vi "generate cartesian circle points.vi"(11 "radius (deg)":dbl=6.0 format="%#_13g") -> (3 "circle XY":cluster{"X[]":dbl[], "Y[]":dbl[]})   [LabVIEW 2017]
doc: "Developed by Kevin Thompson\nkevin@thompsonengineering.net\n\nCopyright 2018-2020\nThompson Engineering, LLC"
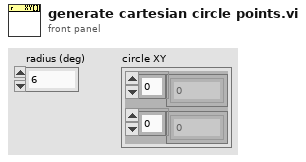
[diagram p1: front panel]
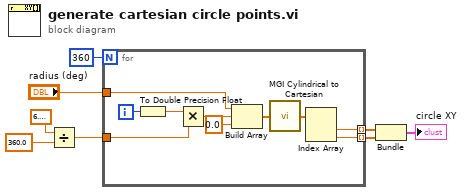
[diagram p0: block diagram]
diagram:
  n1 = Divide(x=6.283185307179586, y=360.0) -> (x/y=w6:dbl)
  n2 = for {
    N: 360 ("degree resolution (360)") -> [_]
    tunnel: [w13] -> w2 mode=indexing
    tunnel: [w12] -> w3 mode=indexing
    tunnel: w6 -> [w11]
    tunnel: "radius (deg)" -> [w10]
    i -> [w9]
    n3 = To Double Precision Float(number=w9) -> (double precision float=w17:dbl)
    n4 = Multiply(x=w17, y=w11) -> (x*y=w16:dbl)
    n5 = Build Array(w10, w16, 0.0 ("element")) -> (w15:dbl[])
    n6 = call <userlib>:"MGI Cylindrical to Cartesian.vi"("R,Th,Z"=w15) -> ("X,Y,Z"=w14:dbl[])
    n7 = Index Array(array=w14) -> (element #1=w13:dbl, element #2=w12:dbl)  [unwired: 2 in]
  }
  n8 = Bundle(w2, w3) -> (→"circle XY":cluster{dbl[], dbl[]})  [unwired: 1 in]
